vi "Write PMUConfigData.vi"(8 "error in (no error)":errorcluster, 10 "PMUConfigData":T1 {"DigitalStatusMask" format="%b"; "Valid Inputs" format="%b"}, 11 "C37.118 PMU in":refnum<class "C37.118 PMU.lvclass">) -> (0 "error out":errorcluster, 3 "C37.118 PMU out":refnum<class "C37.118 PMU.lvclass">)   [LabVIEW 2014, in "SensorPlugins.lvlib" / "C37.118 PMU.lvclass"]
uses:
  C37.118 PMU.lvclass
  Typedef/PMUConfigData.ctl
  Typedef/FormatBits.ctl
  C37.118 PMU.lvclass/C37.118 PMU.ctl
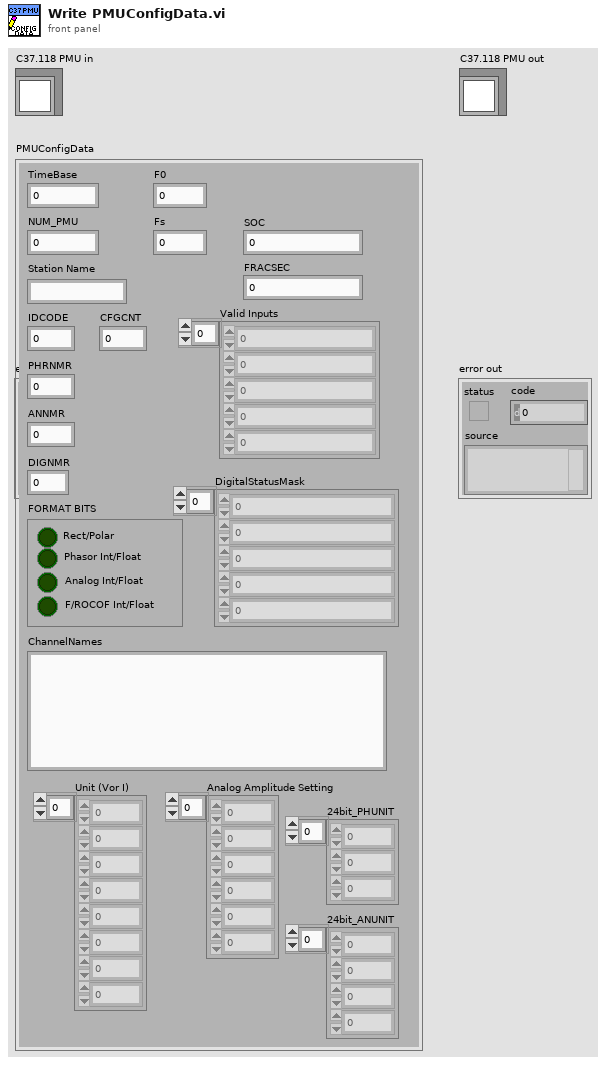
[diagram p1: front panel]
types:
  T1 = typedef "SensorPlugins.lvlib/C37.118 PMU.lvclass/PMUConfigData.ctl" = cluster{"TimeBase":u32, "NUM_PMU":u16, "Station Name":string, "IDCODE":u16, "PHRNMR":u16, "ANNMR":u16, "DIGNMR":u16, "FORMAT BITS":T2, "Valid Inputs":u16[], "DigitalStatusMask":u16[], "24bit_PHUNIT":i32[], "24bit_ANUNIT":u32[], "Analog Amplitude Setting":u32[], "Unit (Vor I)":u8[], "ChannelNames":string, "Fs":i16, "SOC ":u32, "FRACSEC":u32, "F0":sgl, "CFGCNT":u16}
  T2 = typedef "SensorPlugins.lvlib/C37.118 PMU.lvclass/FormatBits.ctl" = cluster{"Rect/Polar":bool, "Phasor Int/Float":bool, "Analog Int/Float":bool, "F/ROCOF Int/Float":bool}
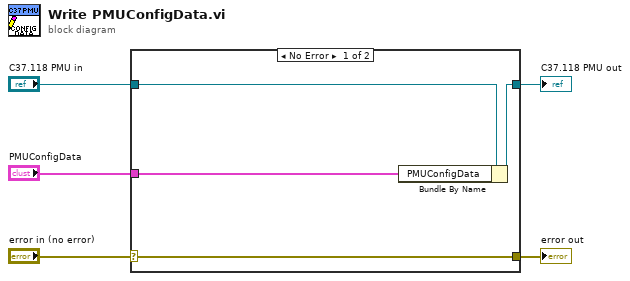
[diagram p0: block diagram]
diagram:
  n1 = case shown="No Error" "error in (no error)" {
    selector: "error in (no error)" -> [w9 w10]
    tunnel: [w9 w10] -> w4
    tunnel: [w7 w11] -> w2
    tunnel: "C37.118 PMU in" -> [w8 w11]
    tunnel: "PMUConfigData" -> [w6 _]
    frame No Error {
      n2 = Bundle By Name(cluster=w8, "PMUConfigData"=w6) -> (w7:refnum<class "C37.118 PMU.lvclass">)
    }
    frame Error {
    }
  }
  "error out" <- w4
  "C37.118 PMU out" <- w2
